vi "test power meter.vi"   [LabVIEW 2018, in "Power Meter.lvlib"]
uses:
  Power Meter.lvlib
  Power Meter/Power Meter.lvclass
  C:/Program Files/National Instruments/LabVIEW 2018/vi.lib/ActorFramework/Actor/Actor.lvclass
  <vilib>/ActorFramework/Message Enqueuer/Message Enqueuer.lvclass/Message Enqueuer.ctl
  <vilib>/ActorFramework/Message Enqueuer/Enqueue.vi
  <vilib>/ActorFramework/Stop Msg/Stop Msg.lvclass
  C:/Program Files/National Instruments/LabVIEW 2018/vi.lib/ActorFramework/Message/Message.lvclass
  <vilib>/ActorFramework/Message Priority Queue/Priority Enqueue.vi
  <vilib>/ActorFramework/Actor/Actor.lvclass
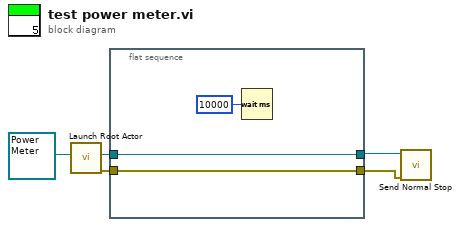
[diagram p0: block diagram]
diagram:
  n1 = call <vilib>:"Launch Root Actor.vi"("Actor"=refnum<class "Power Meter.lvclass"> refnum ("Power Meter.lvlib:Power Meter.lvclass")) -> ("error out"=w3:errorcluster, "Actor's Enqueuer"=w4:refnum<class "Message Enqueuer.lvclass">)  [unwired: 9 in]
  n2 = flat-sequence {
    tunnel: w4 -> [w7]
    tunnel: w3 -> [w8]
    tunnel: [w8] -> w1
    tunnel: [w7] -> w2
    frame #0 {
      n3 = Wait (ms)(milliseconds to wait=u32 10000) -> ()  [unwired: 1 out]
    }
  }
  n4 = call <vilib>:"Send Normal Stop.vi"("error in (no error)"=w1, "Message Enqueuer"=w2) -> ()  [unwired: 9 in, 1 out]
